vi "Recall-Save Memory.vi"(8 "error in (no error)":errorcluster, 9 "Recall/Save (F:Read)":bool, 10 "Memory  (1)":i32=1, 11 "VISA resource name":refnum<visa-resource-name>) -> (0 "error out":errorcluster, 3 "VISA resource name out":refnum<visa-resource-name>)   [LabVIEW 2013, in "Berkeley Nucleonics 500 Series.lvlib"]
doc: "This VI is used to read a previously stored configuration for use or to save the current configuration into one of ten non-volatile memory locations for later use."
uses:
  <instrlib>/Berkeley Nucleonics 500 Series/Berkeley Nucleonics 500 Series.lvlib
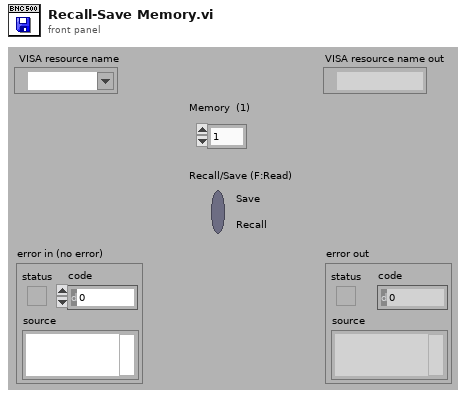
[diagram p1: front panel]
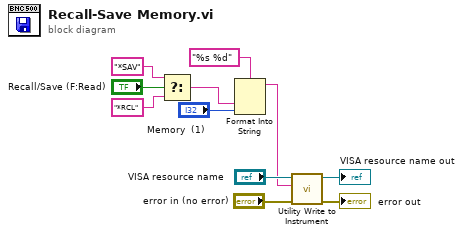
[diagram p0: block diagram]
diagram:
  n1 = Select(t="*SAV", s="Recall/Save (F:Read)", f="*RCL") -> (s? t:f=w5:string)
  n2 = Format Into String(format string="%s %d", w5, "Memory  (1)") -> (resulting string=w7:string)  [unwired: 2 in, 1 out]
  n3 = call <instrlib>:"Utility Write to Instrument.vi"("error in (no error)"="error in (no error)", "Write Buffer"=w7, "VISA resource name"="VISA resource name") -> ("error out"=→"error out":errorcluster, "VISA resource name out"=→"VISA resource name out":refnum<visa-resource-name>)  [unwired: 6 in, 1 out]
